vi "Apply Position To Object.vi"(7 "properties to ignore":variant, 8 "error in (no error)":errorcluster, 9 "scaling settings":T1={"scaling factor"={"horizontal"=1.0, "vertical"=1.0}, "scale text"=FALSE, "scale text position"=FALSE} {"scaling factor"."vertical" min=0.0; "scaling factor"."horizontal" min=0.0}, 10 "GObj Refnum":refnum<vi>, 11 "NI_SE_Object Layout in":refnum<class "Object Layout.lvclass">) -> (0 "error out":errorcluster, 3 "NI_SE_Object Layout out":refnum<class "Object Layout.lvclass">)   [LabVIEW 2010, in "NI_SE_Front Panel Layout.lvlib" / "Object Layout.lvclass"]
uses:
  Object Layout.lvclass
  Scaling Factor_Options.ctl
  XY Scaling Factor.ctl
  Object Layout.lvclass/Object Layout.ctl
  Properties To Ignore.vi
  NI_SE_Front Panel Layout.lvlib
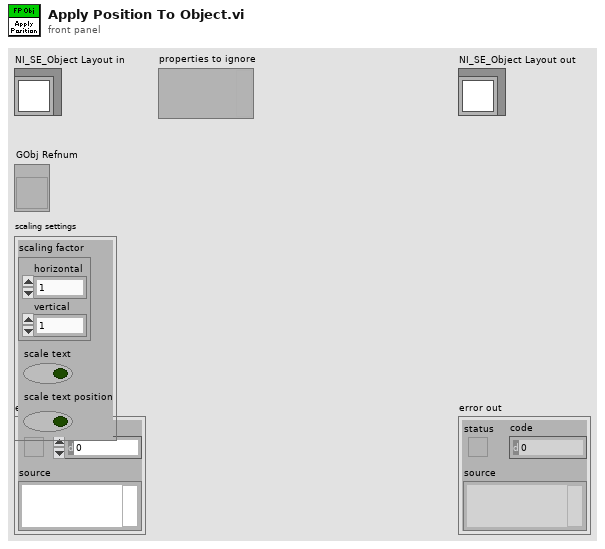
[diagram p1: front panel]
types:
  T1 = typedef "NI_SE_Front Panel Layout.lvlib/Scaling Factor_Options.ctl" = cluster{"scaling factor":T2, "scale text":bool, "scale text position":bool}
  T2 = typedef "NI_SE_Front Panel Layout.lvlib/XY Scaling Factor.ctl" = cluster{"horizontal":dbl, "vertical":dbl}
  T3 = typedef "LVPositionTypeDef.ctl" = cluster{"Left":i32, "Top":i32}
  T4 = typedef "LVRectTypeDef.ctl" = cluster{"left":i16, "top":i16, "right":i16, "bottom":i16}
  T5 = typedef "LVPointTypeDef.ctl" = cluster{"Horizontal":i16, "Vertical":i16}
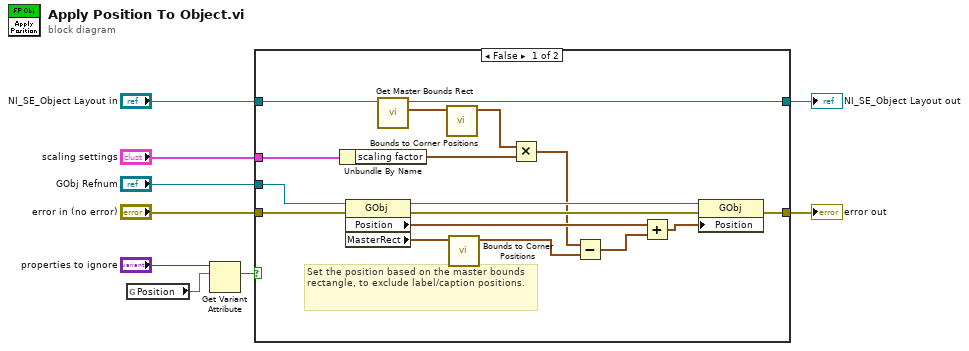
[diagram p0: block diagram]
diagram:
  n1 = global read "Properties To Ignore.vi" "Position"() -> (w1:string)
  n2 = Get Variant Attribute(Variant="properties to ignore", name=w1) -> (found=w3:bool)  [unwired: 2 in, 3 out]
  n3 = case shown="False" w3 {
    tunnel: "error in (no error)" -> [w26 w28]
    tunnel: [w25 w28] -> w8
    tunnel: "NI_SE_Object Layout in" -> [w15 w27]
    tunnel: "scaling settings" -> [w21 _]
    tunnel: "GObj Refnum" -> [w24 _]
    tunnel: [w14 w27] -> w2
    frame False {
      # "Set the position based on the master bounds rectangle, to exclude label/caption positions."
      n4 = Unbundle By Name(w21) -> ("scaling factor"=w19:T2)
      n5 = property class="GObj"(reference=w24, error in=w26) -> (reference out=w22:refnum<vi>, error out=w23:errorcluster, "Position"=w18:T3, "MasterRect"=w11:T4)
      n6 = call "Get Master Bounds Rect.vi"("Object Layout in"=w15) -> ("Rect"=w13:T4, "Object Layout out"=w14:refnum<class "Object Layout.lvclass">)  [unwired: 8 in, 1 out]
      n7 = call "Bounds to Corner Positions.vi"("bounds"=w13) -> ("top left"=w12:T5)  [unwired: 9 in, 1 out]
      n8 = call "Bounds to Corner Positions.vi"("bounds"=w11) -> ("top left"=w10:T5)  [unwired: 9 in, 1 out]
      n9 = Multiply(x=w12, y=w19) -> (x*y=w17:T2)
      n10 = Subtract(x=w17, y=w10) -> (x-y=w20:T2)
      n11 = Add(x=w18, y=w20) -> (x+y=w16:T2)
      n12 = property class="GObj"(reference=w22, error in=w23, "Position"=w16) -> (error out=w25:errorcluster)  [unwired: 1 out]
    }
    frame True {
    }
  }
  "error out" <- w8
  "NI_SE_Object Layout out" <- w2
